vi "build auth URI.vi"(8 "error in (no error)":errorcluster, 10 "State Parameter":string, 11 "Oauth2 in":refnum<class "Oauth2.lvclass">) -> (0 "error out":errorcluster, 2 "Authorization Request URI":string, 3 "Oauth2":refnum<class "Oauth2.lvclass">)   [LabVIEW 2013, in "Oauth2.lvclass"]
uses:
  Oauth2.lvclass
  Oauth2.lvclass/Oauth2.ctl
  <vilib>/LabVIEW Open Source Project/OpenURI/uri/URI.lvclass
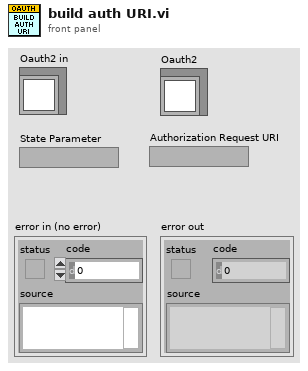
[diagram p1: front panel]
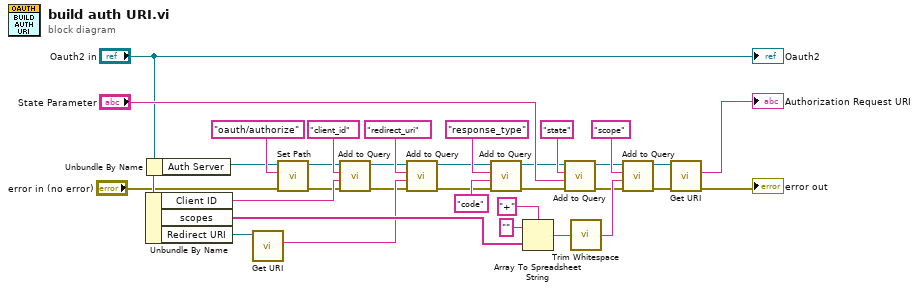
[diagram p0: block diagram]
diagram:
  n1 = Unbundle By Name("Oauth2 in") -> ("Client ID"=w9:string, "scopes"=w32:string[], "Redirect URI"=w33:refnum<class "URI.lvclass">)
  n2 = Unbundle By Name("Oauth2 in") -> ("Auth Server"=w4:refnum<class "URI.lvclass">)
  n3 = call <vilib>:"Get URI.vi"("URI in"=w33) -> ("URI String"=w13:string)  [unwired: 8 in, 2 out]
  n4 = call <vilib>:"Set Path.vi"("error in (no error)"="error in (no error)", "path"="oauth/authorize", "URI in"=w4) -> ("error out"=w7:errorcluster, "URI out"=w6:refnum<class "URI.lvclass">)  [unwired: 7 in]
  n5 = call <vilib>:"Add to Query.vi"("error in (no error)"=w7, "value"=w9, "key"="client_id" ("argument"), "URI in"=w6) -> ("error out"=w10:errorcluster, "URI out"=w11:refnum<class "URI.lvclass">)  [unwired: 6 in]
  n6 = call <vilib>:"Add to Query.vi"("error in (no error)"=w10, "value"=w13, "key"="redirect_uri" ("argument"), "URI in"=w11) -> ("error out"=w14:errorcluster, "URI out"=w15:refnum<class "URI.lvclass">)  [unwired: 6 in]
  n7 = call <vilib>:"Add to Query.vi"("error in (no error)"=w14, "value"="code" ("argument"), "key"="response_type" ("argument"), "URI in"=w15) -> ("error out"=w24:errorcluster, "URI out"=w18:refnum<class "URI.lvclass">)  [unwired: 6 in]
  n8 = Array To Spreadsheet String(delimiter (Tab)="+", array=w32, 3:"" ("format string")) -> (spreadsheet string=w30:string)
  n9 = call <vilib>:"Add to Query.vi"("error in (no error)"=w24, "value"="State Parameter", "key"="state" ("argument"), "URI in"=w18) -> ("error out"=w25:errorcluster, "URI out"=w21:refnum<class "URI.lvclass">)  [unwired: 6 in]
  n10 = call <vilib>:"Trim Whitespace.vi"("string"=w30) -> ("trimmed string"=w31:string)  [unwired: 1 in]
  n11 = call <vilib>:"Add to Query.vi"("error in (no error)"=w25, "value"=w31, "key"="scope" ("argument"), "URI in"=w21) -> ("error out"=w19:errorcluster, "URI out"=w20:refnum<class "URI.lvclass">)  [unwired: 6 in]
  n12 = call <vilib>:"Get URI.vi"("error in (no error)"=w19, "URI in"=w20) -> ("error out"=→"error out":errorcluster, "URI String"=→"Authorization Request URI":string)  [unwired: 7 in, 1 out]
  "Oauth2" <- "Oauth2 in"
